vi "filter tags by seq channel.vi"(9 "exclude? (default: include)":bool, 10 "owner":string, 11 "engine configuration in":refnum<class "base TBM sequencer configuration.lvclass">) -> (2 "seq channel list":refnum<class "TBM channel.lvclass">[](array[class]), 3 "engine configuration out":refnum<class "base TBM sequencer configuration.lvclass">)   [LabVIEW 2014, in "base TBM sequencer configuration.lvclass"]
uses:
  base TBM sequencer configuration.lvclass
  <vilib>/NI/Tag Bus Module Framework/channel/TBM channel.lvclass
  base TBM sequencer configuration.lvclass/base TBM sequencer configuration.ctl
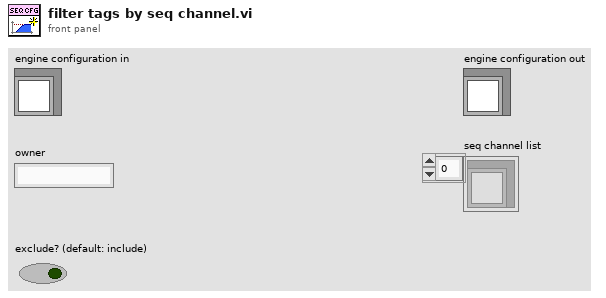
[diagram p1: front panel]
types:
  T1 = typedef "base TBM sequencer configuration.lvclass/Tag Info.ctl" = cluster{"Channel":refnum<class "TBM channel.lvclass">, "Writers":string[], "Readers":string[], "Owning ID":string}
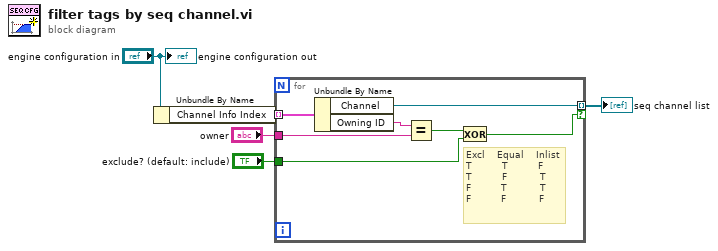
[diagram p0: block diagram]
diagram:
  n1 = Unbundle By Name("engine configuration in") -> ("Channel Info Index"=w4:T1[])
  n2 = for {
    tunnel: w4 -> [w12] mode=indexing
    tunnel: [w11] -> w3 mode=indexing if=w6
    tunnel: "exclude? (default: include)" -> [w7]
    tunnel: "owner" -> [w9]
    # "Excl    Equal    Inlist\nT          T          F \nT          F           T\nF          T           T\nF          F           F"
    n3 = Unbundle By Name(w12) -> ("Channel"=w11:refnum<class "TBM channel.lvclass">, "Owning ID"=w10:string)
    n4 = Equal?(x=w10, y=w9) -> (x = y?=w8:bool)
    n5 = Exclusive Or(1:w7, 2:w8) -> (0:w6:bool)
  }
  "seq channel list" <- w3
  "engine configuration out" <- "engine configuration in"
